vi "pollingOnce.vi"(9 "Rd Deelay":u16=100 max=5000 step=100, 11 "ComPort":refnum<visa-resource-name>="COM10") -> (0 "error out":errorcluster, 1 "Ok":bool, 2 "rssi":i16, 3 "LMS: PID":string)   [LabVIEW 2018]
panel:
  out "Rd Data Size":u16
  out "read butes row":u8[](array[numeric]) format="%x"
  out "received":string
  # "Read TAG"
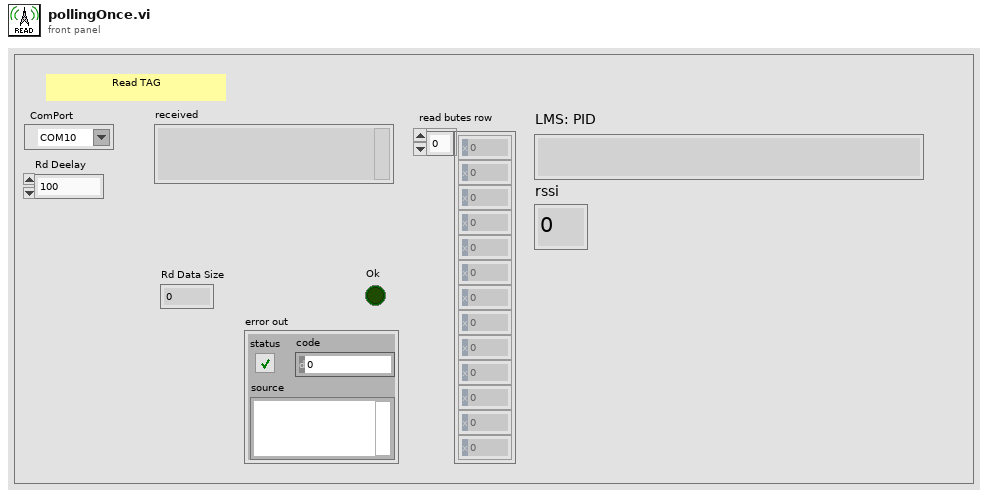
[diagram p1: front panel]
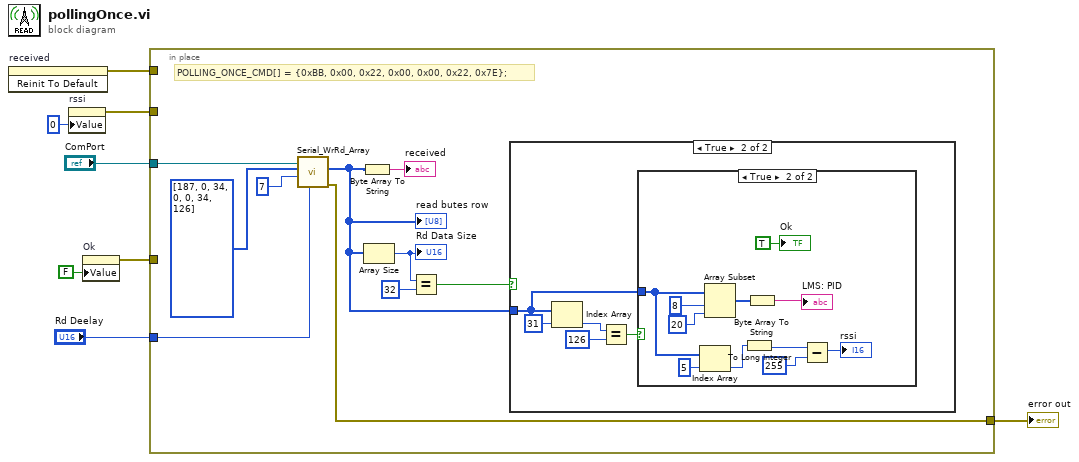
[diagram p0: block diagram]
diagram:
  n1 = invoke on="received" class="Str" method="Reinit To Default"() -> (error out=w6:errorcluster)  [unwired: 3 in, 2 out]
  n2 = property on="rssi" class="DigNum (strict)"("Value"=i16 0 ("rssi")) -> (error out=w4:errorcluster)  [unwired: 2 in, 1 out]
  n3 = property on="Ok" class="Bool (strict)"("Value"=FALSE ("Ok")) -> (error out=w3:errorcluster)  [unwired: 2 in, 1 out]
  n4 = in-place {
    in-place-border: "ComPort" -> [w18]
    in-place-border: "Rd Deelay" -> [w15]
    in-place-border: w6 -> [_]
    in-place-border: w4 -> [_]
    in-place-border: w3 -> [_]
    in-place-border: [w9] -> w1
    # "POLLING_ONCE_CMD[] = {0xBB, 0x00, 0x22, 0x00, 0x00, 0x22, 0x7E};"
    n5 = call "Serial_WrRd_Array.vi"("Read Delay (ms)"=w15, "WR Size"=u16 7, "Array"=u8[] [187, 0, 34, 0, 0, 34, 126], "ComPort"=w18) -> ("error out"=w9:errorcluster, "read butes row"=w11:u8[])  [unwired: 5 in, 1 out]
    "read butes row" <- w11
    n6 = Byte Array To String(unsigned byte array=w11) -> (string=→"received":string)
    n7 = Array Size(array=w11) -> (size(s)=w14:i32)
    "Rd Data Size" <- w14
    n8 = Equal?(x=w14, y=32) -> (x = y?=w12:bool)
    n9 = case shown="True" w12 {
      tunnel: w11 -> [_ w19]
      frame False {
      }
      frame True {
        n10 = Index Array(array=w19, index=31) -> (element=w22:u8)
        n11 = Equal?(x=w22, y=u8 126) -> (x = y?=w20:bool)
        n12 = case shown="True" w20 {
          tunnel: w19 -> [_ w30]
          frame False {
          }
          frame True {
            n13 = Index Array(array=w30, index=5) -> (element=w31:u8)
            n14 = Array Subset(array=w30, index=8, length=20 ("y")) -> (w28:u8[])
            n15 = To Long Integer(number=w31) -> (32bit integer=w33:i32)
            n16 = Byte Array To String(unsigned byte array=w28) -> (string=→"LMS: PID":string)
            n17 = Subtract(x=w33, y=u8 255) -> (x-y=→"rssi":i32)
            "Ok" <- TRUE ("Ok")
          }
        }
      }
    }
  }
  "error out" <- w1
